vi "Fill Menu Rings - LV 2012 NI Verified.vi"() -> ()   [LabVIEW 2012]
panel:
  in  "Array of Menu Rings":u16[](array[ring]) items=["1", "2", "3"]
  in  "Strings to Fill":string[](array[string])
  # "Overview:  Programmatically fills the Menu Ring.\nRequirements: \nLabVIEW 2012 (or compatible).\nInstructions:\n\t1. Fill the String array with the desire data.\n\t2. Run the VI.\n\t3. Check the Ring array to see all the ring elements have the desired data."
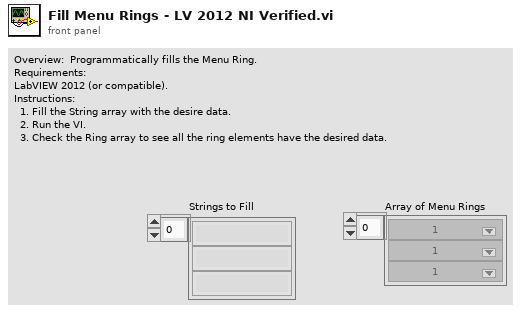
[diagram p1: front panel]
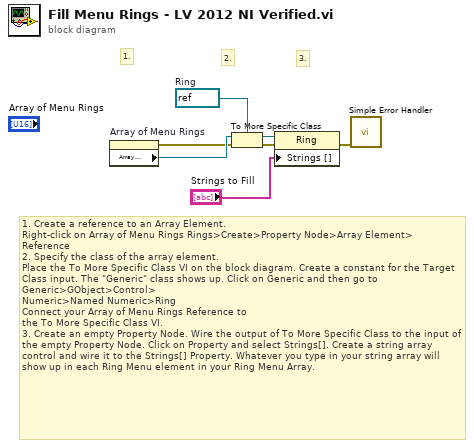
[diagram p0: block diagram]
diagram:
  w7 = refnum<vi> refnum  # Ring
  # "1. Create a reference to an Array Element. \nRight-click on Array of Menu Rings Rings>Create>Property Node>Array Element>\nReference\n2. Specify the class of the array element.\nPlace the To More Specific Class VI on the block diagram. Create a constant for the Target Class input. The \"Generic\" class shows up. Click on Generic and then go to Generic>GObject>Control>\nNumeric>Named Numeric>Ring\nConnect your Array of Menu Rings Reference to \nthe To More Specific Class VI.\n3. Create an empty Property Node. Wire the output of To More Specific Class to the input of the empty Property Node. Click on Property and select Strings[]. Create a string array control and wire it to the Strings[] Property. Whatever you type in your string array will show up in each Ring Menu element in your Ring Menu Array."
  # "3."
  # "2."
  # "1."
  n1 = property on="Array of Menu Rings" class="Arr (strict)"() -> (error out=w5:errorcluster, "Array Element"=w6:refnum<vi>)  [unwired: 2 in, 1 out]
  n2 = To More Specific Class(target class=w7, reference=w6, error in=w5) -> (specific class reference=w4:refnum<vi>, error out=w3:errorcluster)
  n3 = property class="Ring"(reference=w4, error in=w3, "Strings []"="Strings to Fill") -> (error out=w1:errorcluster)  [unwired: 1 out]
  n4 = call <vilib>:"Simple Error Handler.vi"("error in (no error)"=w1) -> ()  [unwired: 4 in, 5 out]
